vi "Get Service Constant.vi"(1 "Service Constant Strings":T1) -> (0 "String Value":string)   [LabVIEW 2019, in "gRPC Template Creation Utility.lvlib"]
uses:
  gRPC Template Creation Utility.lvlib
  ServiceConstants.ctl
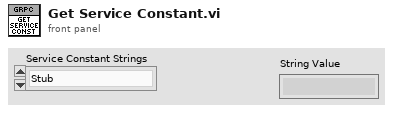
[diagram p1: front panel]
types:
  T1 = typedef "gRPC Template Creation Utility.lvlib/ServiceConstants.ctl" = enum16{"Stub", "Impl", "Usercode_server", "Generated_server", "RPC Service", "RPC Method package_service_method", "ServiceClass out", "ServiceClass in", "RPC Method"}
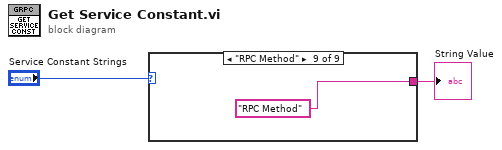
[diagram p0: block diagram]
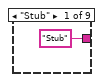
[diagram p2: hidden frame]
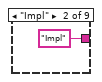
[diagram p3: hidden frame]
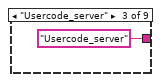
[diagram p4: hidden frame]
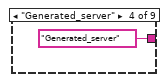
[diagram p5: hidden frame]
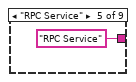
[diagram p6: hidden frame]
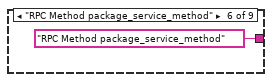
[diagram p7: hidden frame]
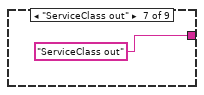
[diagram p8: hidden frame]
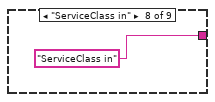
[diagram p9: hidden frame]
diagram:
  n1 = case shown="\"RPC Method\"" "Service Constant Strings" {
    tunnel: ["Stub" "Impl" "Usercode_server" "Generated_server" "RPC Service" "RPC Method package_service_method" "ServiceClass out" "ServiceClass in" "RPC Method"] -> w1
    frame "Stub" {
    }
    frame "Impl" {
    }
    frame "Usercode_server" {
    }
    frame "Generated_server" {
    }
    frame "RPC Service" {
    }
    frame "RPC Method package_service_method" {
    }
    frame "ServiceClass out" {
    }
    frame "ServiceClass in" {
    }
    frame "RPC Method" {
    }
  }
  "String Value" <- w1
